vi "Send Reset Read Statistics.vi"(7 "Message Priority (Normal)":T1=enum."Normal", 8 "error in (no error)":errorcluster, 11 "Message Enqueuer":refnum<class "Message Enqueuer.lvclass">) -> (0 "error out":errorcluster, 3 "Message Enqueuer out":refnum<class "Message Enqueuer.lvclass">)   [LabVIEW 2025, in "Main.lvlib" / "Reset Read Statistics Msg.lvclass"]
doc: "This VI sends the message to an actor."
uses:
  Reset Read Statistics Msg.lvclass
  <vilib>/ActorFramework/Message Enqueuer/Message Enqueuer.lvclass
  <vilib>/ActorFramework/Message Enqueuer/Message Priority.ctl
  C:/Program Files/National Instruments/LabVIEW 2025/vi.lib/ActorFramework/Message/Message.lvclass
  <vilib>/ActorFramework/Message Enqueuer/Message Enqueuer.lvclass/Message Enqueuer.ctl
  <vilib>/ActorFramework/Message Priority Queue/Priority Enqueue.vi
  Reset Read Statistics Msg.lvclass/Reset Read Statistics Msg.ctl
  C:/Users/natan/Documents/Flash me if you can/Main/Main Messages/Reset Read Statistics Msg/Reset Read Statistics Msg.lvclass
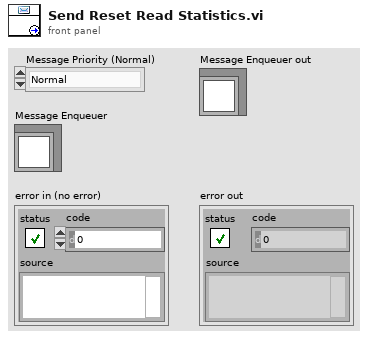
[diagram p1: front panel]
types:
  T1 = typedef "Actor Framework.lvlib/Message Enqueuer.lvclass/Message Priority.ctl" = enum16{"Low", "Normal", "High"}
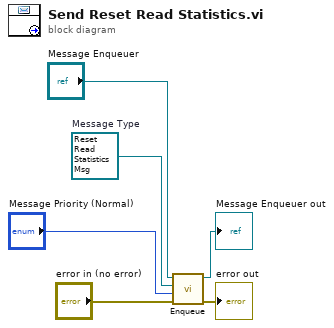
[diagram p0: block diagram]
diagram:
  w3 = refnum<class "Reset Read Statistics Msg.lvclass"> refnum  # Message Type
  n1 = call <vilib>:"Enqueue.vi"("error in (no error)"="error in (no error)", "Message Priority (Normal)"="Message Priority (Normal)", "Message"=w3, "Message Enqueuer in"="Message Enqueuer") -> ("error out"=→"error out":errorcluster, "Message Enqueuer out"=→"Message Enqueuer out":refnum<class "Message Enqueuer.lvclass">)  [unwired: 6 in]
